vi "Untitled 5.vi"() -> ()   [LabVIEW 2010]
uses:
  <instrlib>/Fluke 2625A/Fluke 2625A.lvlib
panel:
  in  "VISA resource name 3":refnum<visa-resource-name>
  out "read buffer 3":string
  out "error out 3":errorcluster
  out "read buffer 2":string
  out "read buffer":string
  out "return count 2":u32
  in  "VISA resource name 2":refnum<visa-resource-name>
  out "error out 2":errorcluster
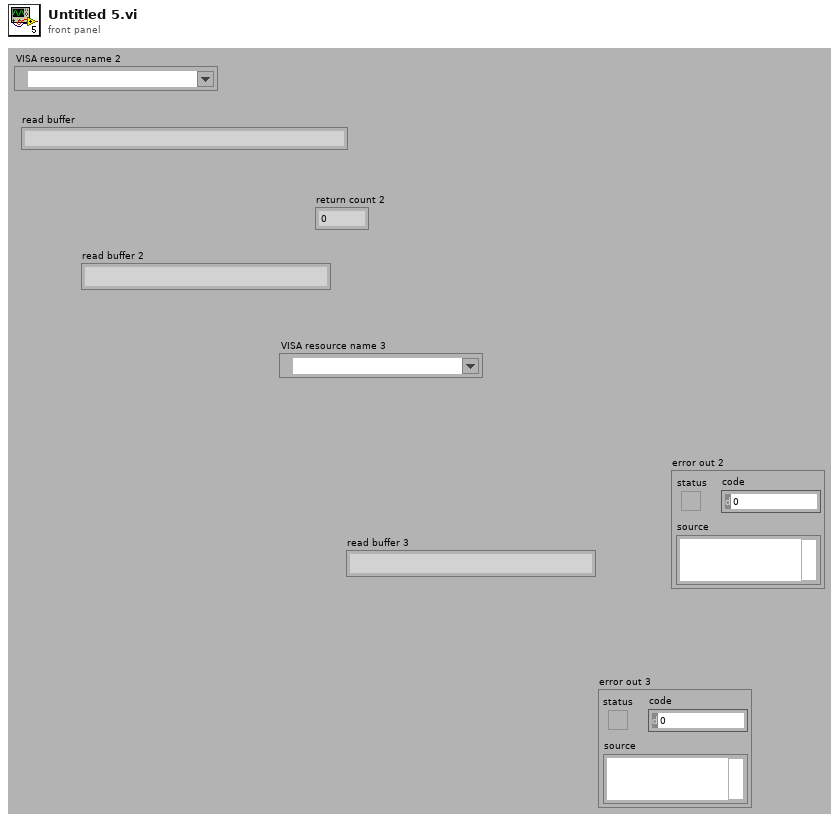
[diagram p1: front panel]
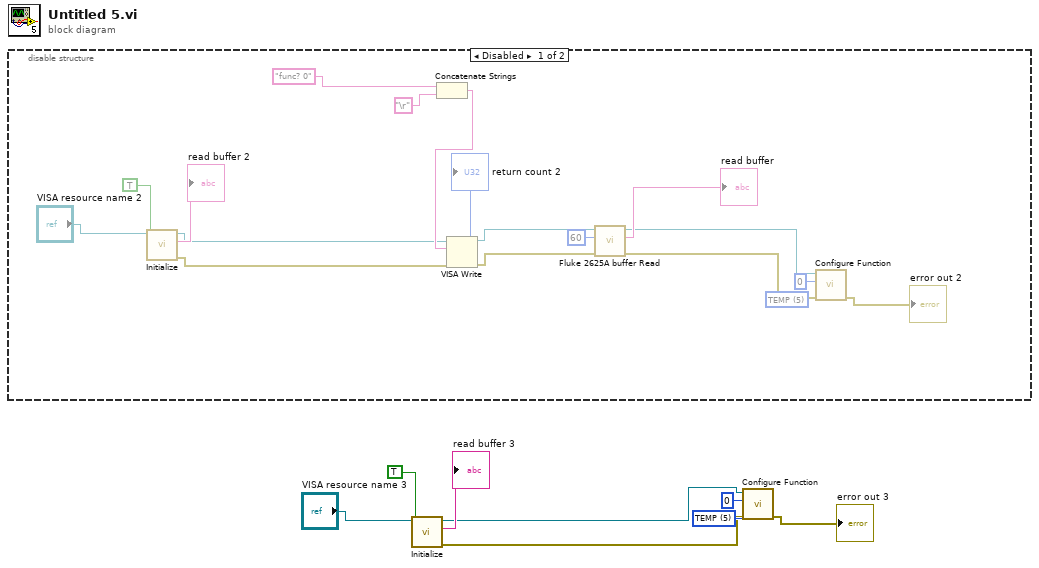
[diagram p0: block diagram]
diagram:
  w8 = u16 5 items=["OFF", "VDC", "VAC", "OHMS", "FREQ", "TEMP"] ("Function (5: Temp)")
  n1 = disable-structure shown="Disabled" {
    frame Disabled {
      w9 = u16 5 items=["OFF", "VDC", "VAC", "OHMS", "FREQ", "TEMP"] ("Function (5: Temp)")
      n2 = call <instrlib>:"Initialize.vi"(9:TRUE, "VISA resource name"="VISA resource name 2") -> ("error out"=w14:errorcluster, "read buffer"=→"read buffer 2":string, "VISA resource name out"=w15:refnum<visa-resource-name>)  [unwired: 7 in]
      n3 = Concatenate Strings("func? 0" ("write buffer"), "\r") -> (w21:string)
      n4 = VISA Write(VISA resource name=w15, write buffer=w21, error in (no error)=w14) -> (VISA resource name out=w20:refnum<visa-resource-name>, return count=→"return count 2":u32, error out=w19:errorcluster)
      n5 = call <instrlib>:"Fluke 2625A buffer Read.vi"("error out"=w19, "byte count"=u32 60, "VISA resource name out"=w20) -> ("error out 2"=w12:errorcluster, "read buffer"=→"read buffer":string, "VISA resource name out 2"=w13:refnum<visa-resource-name>)  [unwired: 6 in]
      n6 = call <instrlib>:"Configure Function.vi"("error in (no error)"=w12, "Resistance (0: 300 Ohms)  2"=w9, "Frequency (0: 900 Hz)"=i8 0 ("Channel"), "VISA resource name"=w13) -> ("error out"=→"error out 2":errorcluster)  [unwired: 5 in, 1 out]
    }
    frame Enabled {
    }
  }
  n7 = call <instrlib>:"Initialize.vi"(9:TRUE, "VISA resource name"="VISA resource name 3") -> ("error out"=w1:errorcluster, "read buffer"=→"read buffer 3":string, "VISA resource name out"=w2:refnum<visa-resource-name>)  [unwired: 7 in]
  n8 = call <instrlib>:"Configure Function.vi"("error in (no error)"=w1, "Resistance (0: 300 Ohms)  2"=w8, "Frequency (0: 900 Hz)"=i8 0 ("Channel"), "VISA resource name"=w2) -> ("error out"=→"error out 3":errorcluster)  [unwired: 5 in, 1 out]
